vi "SR Scan.vi"() -> ()   [LabVIEW 2014]
uses:
  user.lib/SpectralRadar.llb/LabVIEW Helper.lvlib
  <vilib>/Utility/error.llb/DialogType.ctl
  user.lib/SpectralRadar.llb/OCT Device.lvclass
  user.lib/SpectralRadar.llb/Processing.lvclass
  user.lib/SpectralRadar.llb/Probe.lvclass
  user.lib/SpectralRadar.llb/FullRange.lvclass
  user.lib/SpectralRadar.llb/Settings.lvclass
  user.lib/SpectralRadar.llb/FileSelection.lvlib
  user.lib/SpectralRadar.llb/Scan Pattern.lvclass
  user.lib/SpectralRadar.llb/Raw Data.lvclass
  user.lib/SpectralRadar.llb/Data.lvclass
  user.lib/SpectralRadar.llb/display Data 1D in XY-Graph.vi
  user.lib/SpectralRadar.llb/Normal Direction Selection.ctl
  user.lib/SpectralRadar.llb/Colored Data.lvclass
  user.lib/SpectralRadar.llb/Buffer.lvclass
  user.lib/SpectralRadar.llb/Coloring.lvclass
  user.lib/SpectralRadar.llb/Colored Data Export Format Selection.ctl
  user.lib/SpectralRadar.llb/Probe Parameter Int Selection.ctl
  user.lib/SpectralRadar.llb/Processing Parameter Int Selection.ctl
  user.lib/SpectralRadar.llb/ImageField.lvclass
  user.lib/SpectralRadar.llb/display Data 2D.vi
  user.lib/SpectralRadar.llb/Post Processing.lvlib
  user.lib/SpectralRadar.llb/Raw Data Export Format Selection.ctl
  user.lib/SpectralRadar.llb/Data Analyzation Selection.ctl
  user.lib/SpectralRadar.llb/Coloring Byteorder.ctl
  user.lib/SpectralRadar.llb/set Scan Output.vi
  user.lib/SpectralRadar.llb/Data Export Format Selection.ctl
  user.lib/SpectralRadar.llb/Colorscheme Selection.ctl
panel:
  in  "Average A-scan":bool
  in  "Boolean 2":bool
  in  "Filter Options":bool
  in  "Filter":bool
  in  "B-Scan \nAveraging":i32=1 min=1 max=20 step=1
  in  "BScan angle \n[deg]":dbl(knob) scale=0.0..180.0 scale format="%#.6g"
  in  "BScan\nY offset [mm]":dbl min=-5.0 max=5.0 format="%_4f"
  in  "BScan\nX offset [mm]":dbl min=-5.0 max=5.0 format="%_4f"
  out "ImageField":refnum<class "ImageField.lvclass">
  in  "Auto Range Button":bool
  in  "Image field correction":bool
  out "Save All Progress":i32(slide) min=0 max=35 scale=0.0..11.0
  in  "Palette":T1
  in  "Light":dbl(slide)=51.27999885380268 caption="Sharpness" min=0.0 max=100.0 step=0.009999999776482582 scale=0.0..100.0
  out "Coloring":refnum<class "Coloring.lvclass">
  out "GalvoControl":refnum<class "Probe.lvclass">
  out "Scan Pattern":refnum<class "Scan Pattern.lvclass">
  out "AutoSafe":bool
  in  "Stability":dbl(slide) caption="SNR" min=0.0 max=1.0 step=1.0
  in  "Averaging*Binning":i32(slide)=1 caption="Quality" min=1 max=200 step=1 scale=1.0..200.0
  in  "Options":bool
  in  "Window":T2(ring)
  in  "ShowVideoImage":bool=TRUE caption="Show Video Image"
  out "StreamingPath":path
  in  "Streaming":bool caption="Stream B-Scans"
  out "Image":T3(plugin-control)
  out "Frame Rate":dbl=6.134969234466553 format="%#_3g"
  in  "RunMeasurement":bool
  out "StopIndicator":bool
  in  "Save all":bool
  in  "Brightness":sgl(slide)=0.5272727 caption="Sharpness" min=0 max=1 step=0.01 scale=0.0..1.0
  in  "Contrast":sgl(slide)=0.53333336 caption="Sharpness" min=0 max=1 step=0.01 scale=0.0..1.0
  in  "Saturation":sgl(slide)=0.5212121 caption="Sharpness" min=0 max=1 step=0.01 scale=0.0..1.0
  out "Spacing Z":dbl=2.0 min=1.0 max=500.0 step=1.0 format="%-#2_3f"
  in  "Save":bool
  in  "Description":string
  in  "LowerBScanBorder":dbl=0.972000002861023 min=1.4420210526315789 max=4.806736842105263 step=0.1 format="%.2f"
  in  "UpperBScanBorder":dbl min=0.0 max=0.9613473684210526 step=0.10000000149011612 format="%.2f"
  out "Reference Intensity":sgl(slide) max=140000 scale=0.0..1.0
  out "Next File Name":path=path "D:/OCTData"
  in  "Set Path":bool
  in  "Recallibrate":bool
  in  "Range X [mm]":dbl=2.0 caption="Bereich [mm]" min=0.0 max=10.0 step=0.5 format="%_3f"
  out "Spacing X [µm]":dbl=2.0 min=1.0 max=500.0 step=1.0 format="%#_3g"
  in  "Columns":i32=1000 min=50 max=10240 step=1
  in  "Cursors":bool
  out "Cursor on":bool
  in  "Index of Refraction":dbl=1.0 min=1.0 max=5.0 step=0.10000000149011612 format="%.3f"
  out "Distance Y [mm]":sgl format="%.3f"
  out "Distance X [mm]":sgl format="%.3f"
  out "AScan":cluster{"B-Scan":sgl[], i32[]}(graph)
  in  "Image#":i32=1 caption="of 0" min=1 max=1 step=1
  in  "QuitApp":bool
  in  "Boundries":cluster{sgl, sgl}(slide)={76.65738, 42.00557} scale=15.0..120.0
  out "B-Scan":sgl[][](graph)
  # "Version 5.0"
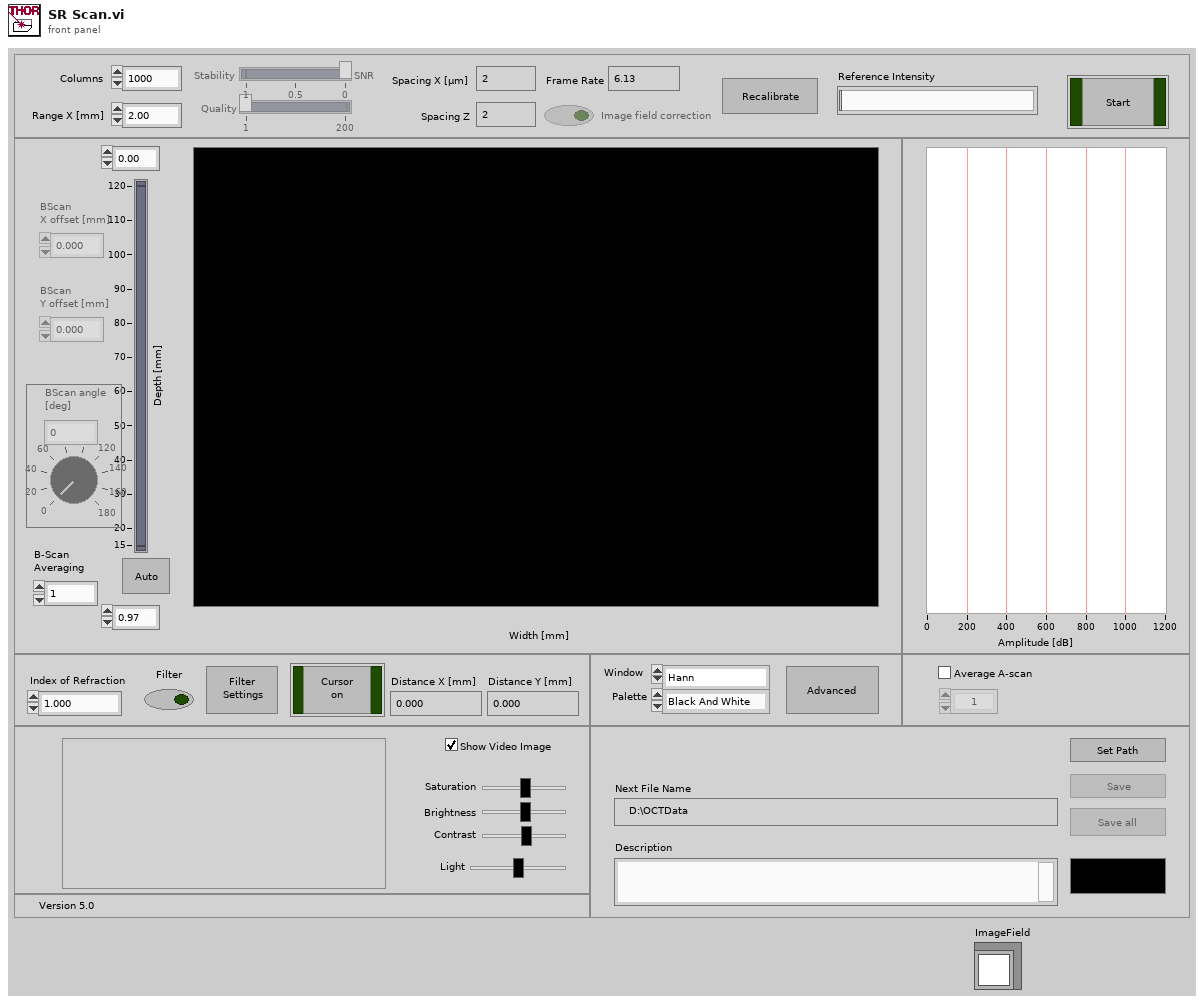
[diagram p1: front panel]
types:
  T1 = typedef "Coloring.lvclass/Colorscheme Selection.ctl" = enum16{"Black And White", "Inverted Black And White", "Color", "Black and Orange", "Black and Red", "Doppler Phase Coloring"}
  T2 = enum16{"Hann", "Hamming", "Gauss", "Tapered Cosine", "Blackman", "4 Term B-Harris"}
  T3 = typedef "IMAQ Image.ctl" = refnum<image>
  T4 = typedef "Coloring.lvclass/Coloring Byteorder.ctl" = enum16{"RGBA32", "BGRA32", "ARGB32", ""}
  T5 = enum16{"Full Well Capacity", "z Spacing", "z Range", "Dynamc Range Min [dB]", "Dynamic Range Low [dB]", "Dynamic Range High [dB]", "Dynamic Range Max [dB]"}
  T6 = typedef "Probe.lvclass/Probe Parameter Int Selection.ctl" = enum16{"Apodization Cycles", "Oversampling", "Oversampling Slow Axis", "Speckle Reduction"}
  T7 = typedef "Processing.lvclass/Processing Parameter Int Selection.ctl" = enum32{"Spectrum Averaging", "A-Scan Averaging", "B-Scan Averaging", "Zero Padding", "Number of Threads", "Fourier Averaging"}
  T8 = typedef "Data.lvclass/Normal Direction Selection.ctl" = enum16{"Direction 1", "Direction 2", "Direction 3"}
  T9 = typedef "Data.lvclass/Data Export Format Selection.ctl" = enum16{"SRM (Spectral Radar Metafile)", "RAW", "CSV", "TXT", "Table TXT", "Fits", "VFF", "VTK", "TIFF"}
  T10 = typedef "Colored Data.lvclass/Colored Data Export Format Selection.ctl" = enum16{"SRM (Spectral Radar Metafile)", "RAW", "BMP", "PNG", "JPG", "PDF", "TIFF"}
  T11 = enum16{"Asynchronous Continuous", "Asynchronous Finite", "Synchronous"}
  T12 = typedef "Data.lvclass/Data Analyzation Selection.ctl" = enum16{"Min", "Mean", "Max"}
  T13 = typedef "Raw Data.lvclass/Raw Data Export Format Selection.ctl" = enum16{"RAW", "SRR (Spectral Radar Raw)"}
  T14 = typedef "DialogType.ctl" = u16
  T15 = typedef "Image Type" = u32
  T16 = enum8{"Enabled", "Disabled", "Disabled and Grayed Out"}
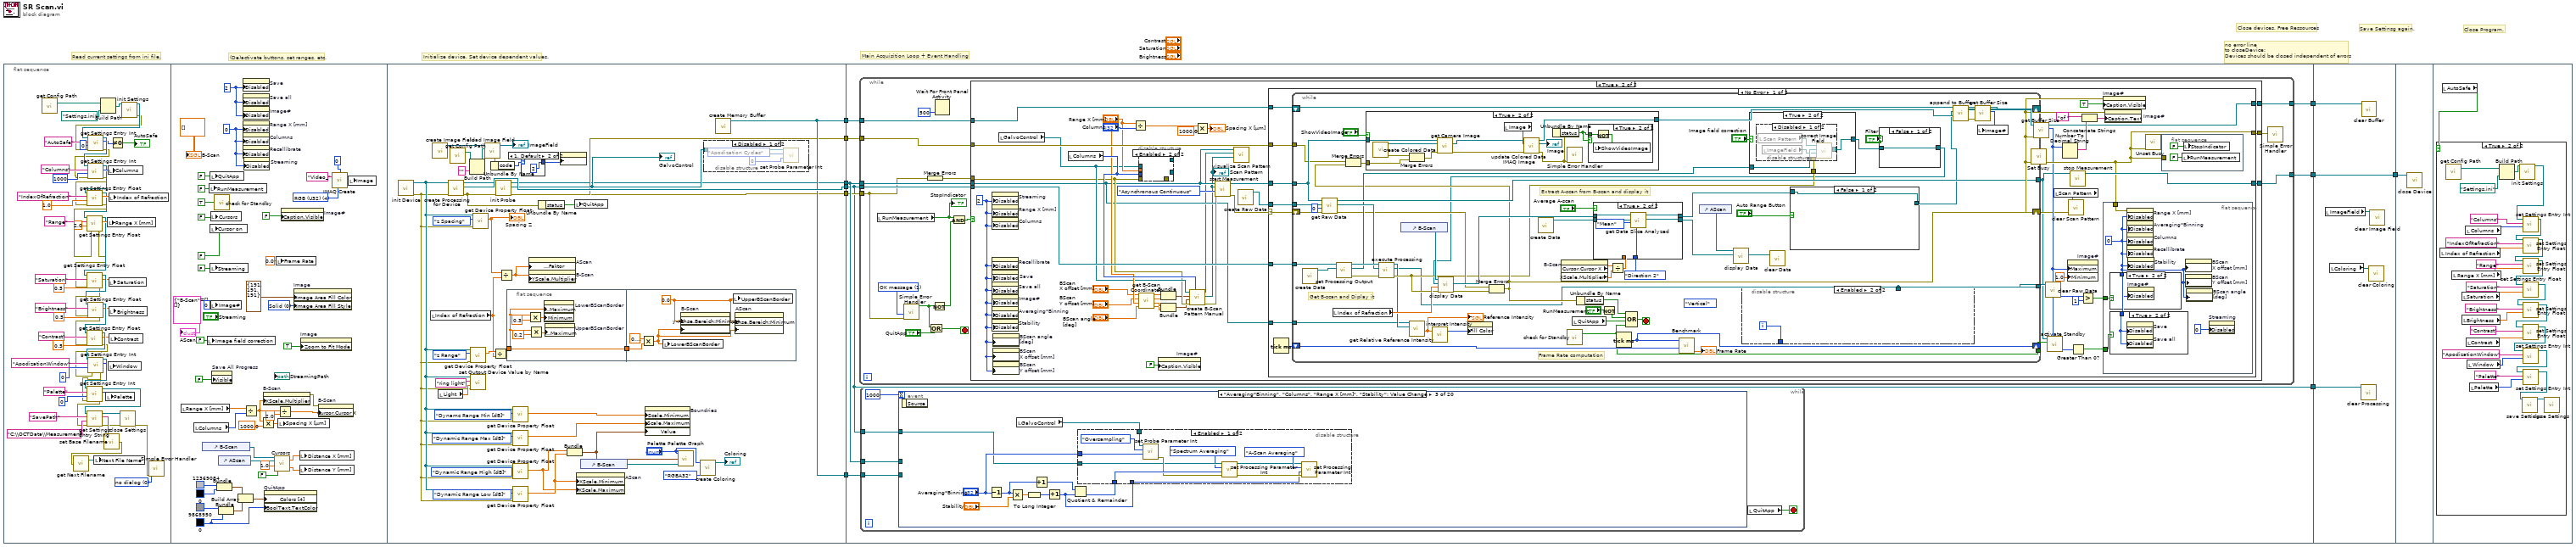
[diagram p0: block diagram]
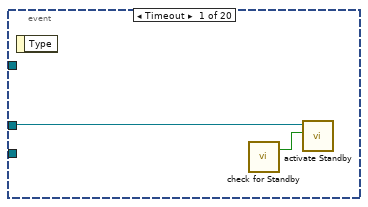
[diagram p4: hidden frame]
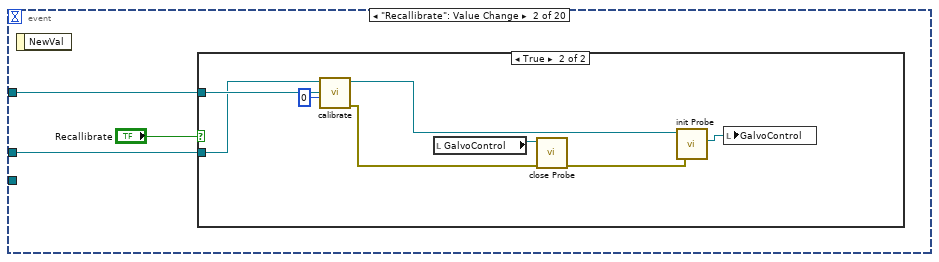
[diagram p5: hidden frame]
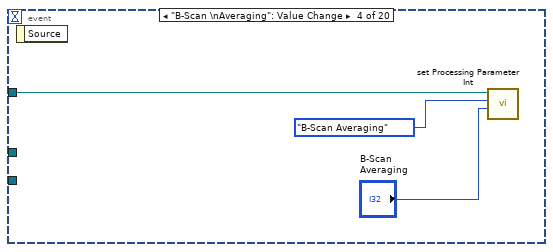
[diagram p8: hidden frame]
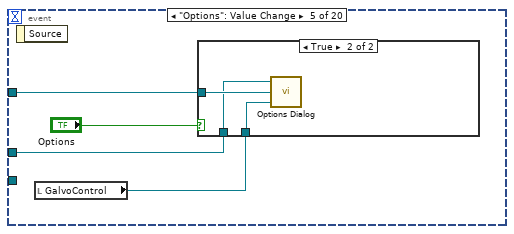
[diagram p9: hidden frame]
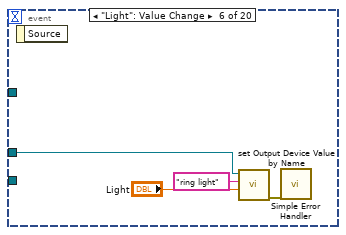
[diagram p11: hidden frame]
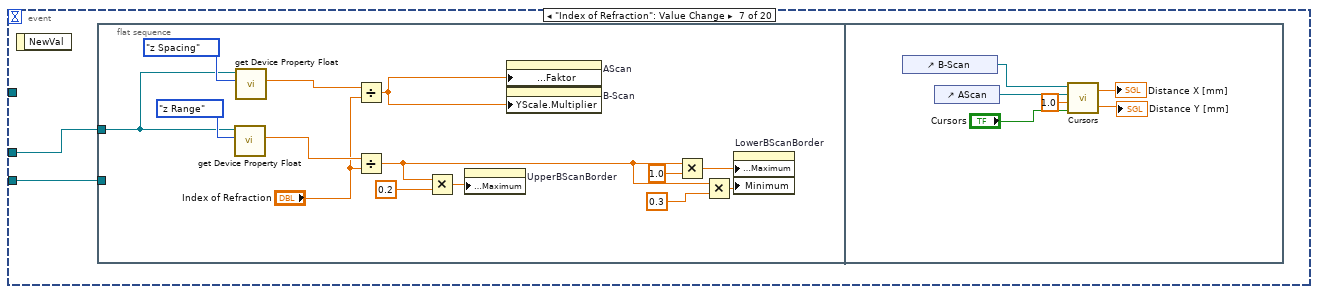
[diagram p12: hidden frame]
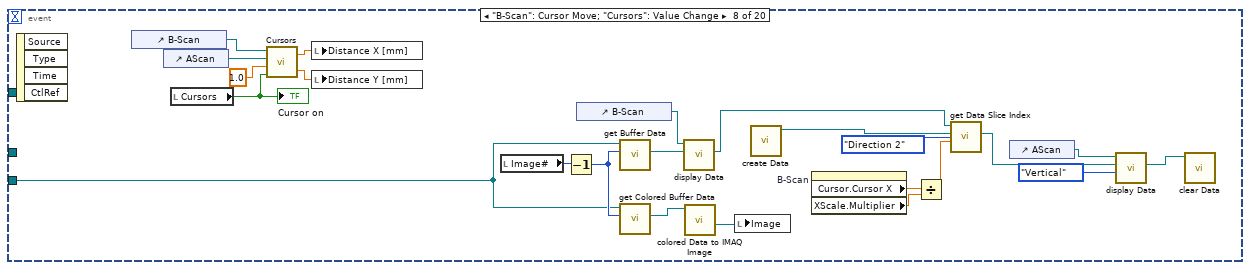
[diagram p13: hidden frame]
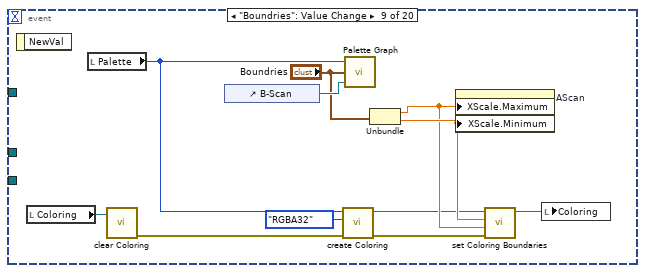
[diagram p14: hidden frame]
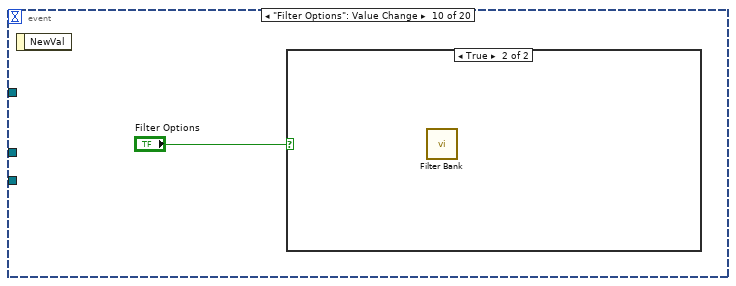
[diagram p15: hidden frame]
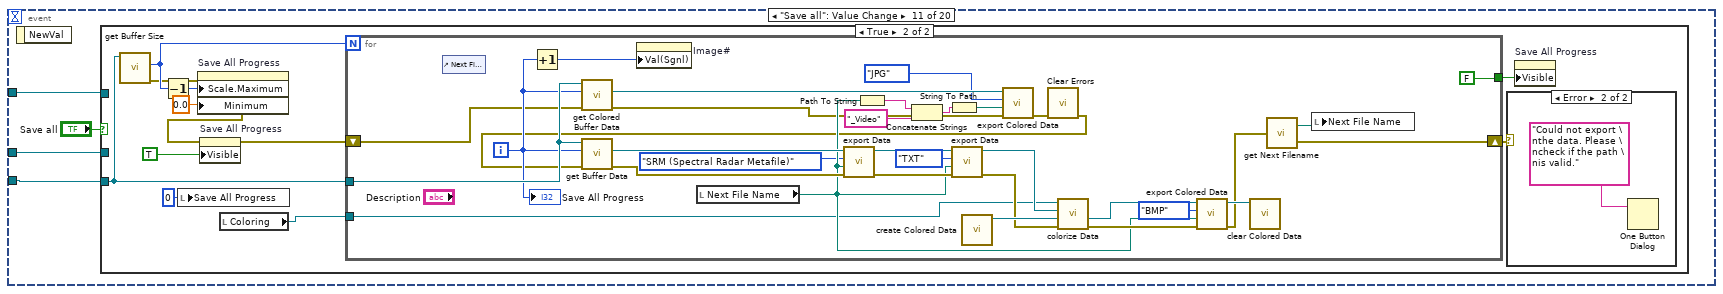
[diagram p17: hidden frame]
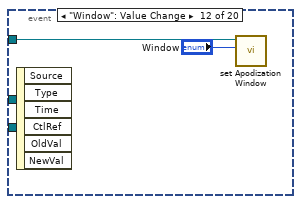
[diagram p20: hidden frame]
diagram:
  # "Close Program."
  # "Save Settinsg again."
  # "Close devices, Free Ressources"
  # "Main Acquisition Loop + Event Handling"
  # "Initialize device. Set device dependent values."
  # "(De)activate buttons, set ranges, etc."
  # "Read current settings from ini file."
  # "no error line\nto closeDevice:\nDevices should be closed independent of errors"
  n1 = flat-sequence {
    tunnel: [w114] -> w10
    tunnel: [w116] -> w7
    tunnel: [w151] -> w6
    tunnel: [w115] -> w4
    tunnel: [w140] -> w3
    tunnel: [w140] -> w1
    tunnel: w10 -> [w175]
    tunnel: [w176] -> w8
    tunnel: w7 -> [w174]
    tunnel: w6 -> [w172]
    tunnel: [w172] -> w5
    tunnel: w4 -> [w173]
    tunnel: w3 -> [w171]
    tunnel: [w170] -> w2
    tunnel: w1 -> [w169]
    tunnel: [w668] -> w9
    tunnel: w8 -> [w668]
    tunnel: w5 -> [w667]
    tunnel: w2 -> [w666]
    tunnel: w9 -> [w669]
    frame #0 {
      w22 = T14 0 items=["no dialog", "OK message", "continue or stop message", "OK message + warnings", "continue/stop + warnings"] ("type of dialog (OK msg:1)")
      n2 = call "get Config Path.vi"() -> ("Path"=w25:path)  [unwired: 1 in, 1 out]
      n3 = Build Path(base path=w25, name or relative path=path "Settings.ini" ("Relative \"SpectralRadar.ini\" Path")) -> (appended path=w69:path)
      n4 = call "init Settings.vi"("Path to settings file"=w69) -> ("error out"=w24:errorcluster, "Settings"=w56:refnum<class "Settings.lvclass">)  [unwired: 5 in]
      n5 = call "get Settings Entry Int.vi"("error in (no error)"=w24, "Default Value"=0, "Node Name"="AutoSafe", "Settings"=w56) -> ("error out"=w19:errorcluster, "Value"=w53:i32, "Settings"=w57:refnum<class "Settings.lvclass">)  [unwired: 1 in]
      n6 = call "get Settings Entry Int.vi"("error in (no error)"=w19, "Default Value"=1000, "Node Name"="Columns", "Settings"=w57) -> ("error out"=w18:errorcluster, "Value"=w67:i32, "Settings"=w59:refnum<class "Settings.lvclass">)  [unwired: 1 in]
      n7 = call "get Settings Entry Float.vi"("error in (no error)"=w18, "Default Value"=1.0, "Node Name"="IndexOfRefraction", "Settings"=w59) -> ("error out"=w17:errorcluster, "Value"=w63:dbl, "Settings"=w58:refnum<class "Settings.lvclass">)  [unwired: 1 in]
      n8 = call "get Settings Entry Float.vi"("error in (no error)"=w17, "Default Value"=2.0, "Node Name"="Range", "Settings"=w58) -> ("error out"=w16:errorcluster, "Value"=w60:dbl, "Settings"=w49:refnum<class "Settings.lvclass">)  [unwired: 1 in]
      n9 = call "get Settings Entry Float.vi"("error in (no error)"=w16, "Default Value"=0.5, "Node Name"="Saturation", "Settings"=w49) -> ("error out"=w15:errorcluster, "Value"=w35:dbl, "Settings"=w46:refnum<class "Settings.lvclass">)  [unwired: 1 in]
      n10 = call "get Settings Entry Float.vi"("error in (no error)"=w15, "Default Value"=0.5, "Node Name"="Brightness", "Settings"=w46) -> ("error out"=w14:errorcluster, "Value"=w34:dbl, "Settings"=w39:refnum<class "Settings.lvclass">)  [unwired: 1 in]
      n11 = call "get Settings Entry Float.vi"("error in (no error)"=w14, "Default Value"=0.5, "Node Name"="Contrast", "Settings"=w39) -> ("error out"=w13:errorcluster, "Value"=w33:dbl, "Settings"=w38:refnum<class "Settings.lvclass">)  [unwired: 1 in]
      n12 = call "get Settings Entry Int.vi"("error in (no error)"=w13, "Default Value"=0, "Node Name"="ApodizationWindow", "Settings"=w38) -> ("error out"=w12:errorcluster, "Value"=w36:i32, "Settings"=w37:refnum<class "Settings.lvclass">)  [unwired: 1 in]
      n13 = call "get Settings Entry Int.vi"("error in (no error)"=w12, "Default Value"=0, "Node Name"="Palette", "Settings"=w37) -> ("error out"=w11:errorcluster, "Value"=w20:i32, "Settings"=w31:refnum<class "Settings.lvclass">)  [unwired: 1 in]
      n14 = call "get Settings Entry String.vi"("error in (no error)"=w11, "Default Value"="C:\\OCTData\\Measurement", "Node Name"="SavePath", "Settings"=w31) -> ("error out"=w23:errorcluster, "Value"=w28:string, "Settings"=w30:refnum<class "Settings.lvclass">)  [unwired: 1 in]
      n15 = call "set Base Filename.vi"("Base"=w28) -> ("error out"=w27:errorcluster)  [unwired: 1 in]
      n16 = call "get Next Filename.vi"("error in (no error)"=w27) -> ("Next File Name"=w26:path)  [unwired: 1 out]
      n17 = local write "Next File Name"(w26) -> ()
      n18 = local write "Palette"(w20) -> ()
      n19 = local write "Range X [mm]"(w60) -> ()
      n20 = local write "Columns"(w67) -> ()
      n21 = local write "Window"(w36) -> ()
      n22 = local write "Index of Refraction"(w63) -> ()
      n23 = local write "Saturation"(w35) -> ()
      n24 = local write "Brightness"(w34) -> ()
      n25 = local write "Contrast"(w33) -> ()
      n26 = Not Equal To 0?(x=w53) -> (x != 0?=→"AutoSafe":bool)
      n27 = call "close Settings.vi"("error in (no error)"=w23, "Settings"=w30) -> ("error out"=w21:errorcluster)  [unwired: 5 in]
      n28 = call <vilib>:"Simple Error Handler.vi"("type of dialog (OK msg:1)"=w22, "error in (no error)"=w21) -> ()  [unwired: 3 in, 5 out]
    }
    frame #1 {
      w77 = T15 4 items=["Grayscale (U8)", "Grayscale (I16)", "Grayscale (SGL)", "Complex (CSG)", "RGB (U32)", "HSL (U32)", "RGB (U64)", "Grayscale (U16)"] ("Image Type")
      w83 = u32 0 items=["Default"=3, "Solid"=0, "Hatch"=2] ("Image Area:Background:Fill Style")
      w104 = u32 0
      w112 = u8 0 ("Deaktiviert")
      w113 = u8 2 ("Deaktiviert")
      n29 = local read "Range X [mm]"() -> (w90:dbl)
      n30 = local read "Columns"() -> (w85:i32)
      n31 = control-ref of="B-Scan"() -> (w93:refnum<vi>)
      n32 = local write "Image field correction"(FALSE ("Confocal correction")) -> ()
      n33 = local write "RunMeasurement"(FALSE ("s/t")) -> ()
      n34 = local write "QuitApp"(FALSE ("QuitApp")) -> ()
      n35 = local write "Cursor on"(FALSE ("Cursor on")) -> ()
      n36 = local write "Streaming"(FALSE ("Streaming")) -> ()
      n37 = local write "Cursors"(FALSE ("Cursors")) -> ()
      n38 = local write "Image#"(0 ("Image#")) -> ()
      n39 = property on="Save All Progress" class="Slide (strict)"("Visible"=FALSE) -> ()  [unwired: 2 in, 2 out]
      n40 = call "check for Standby.vi"("ResetTimer"=TRUE) -> ()  [unwired: 2 out]
      n41 = Bundle(u32 12369084, u32 0) -> (w101:cluster{u32, u32})  [unwired: 1 in]
      n42 = control-ref of="AScan"() -> (w94:refnum<vi>)
      n43 = Bundle(u32 9868950, w104) -> (w102:cluster{u32, u32})  [unwired: 1 in]
      n44 = Build Array(w101, w102) -> (w103:cluster{u32, u32}[])
      n45 = property on="Save" class="Bool"("Disabled"=w113) -> ()  [unwired: 2 in, 2 out]
      n46 = property on="Save all" class="Bool (strict)"("Disabled"=w113) -> ()  [unwired: 2 in, 2 out]
      n47 = property on="Image#" class="DigNum (strict)"("Disabled"=w113) -> ()  [unwired: 2 in, 2 out]
      n48 = property on="Range X [mm]" class="DigNum (strict)"("Disabled"=w112) -> ()  [unwired: 2 in, 2 out]
      n49 = property on="Columns" class="DigNum (strict)"("Disabled"=w112) -> ()  [unwired: 2 in, 2 out]
      n50 = property on="Recallibrate" class="Bool"("Disabled"=w112) -> ()  [unwired: 2 in, 2 out]
      n51 = property on="Streaming" class="Bool (strict)"("Disabled"=w112) -> ()  [unwired: 2 in, 2 out]
      n52 = Divide(x=w90, y=w85) -> (x/y=w88:dbl)
      n53 = Multiply(x=w88, y=1000.0) -> (x*y=w86:dbl)
      n54 = property on="B-Scan" class="IntGraph (strict)"("XScale.Multiplier"=w88) -> (error out=w91:errorcluster)  [unwired: 2 in, 1 out]
      n55 = property on="QuitApp" class="Bool (strict)"("Colors [4]"=w103, "BoolText.TextColor"=w104) -> ()  [unwired: 2 in, 2 out]
      n56 = call "Cursors.vi"("Cursors"=FALSE, "IndexOfRefraction"=sgl 1.0, "ReferenceAScan"=w94, "ReferenceBScan"=w93) -> ("DistanceZ"=w97:sgl, "DistanceX"=w96:sgl)
      n57 = local write "Frame Rate"(0.0 ("Frame Rate")) -> ()
      n58 = Divide(x=w88, y=2.0) -> (x/y=w87:dbl)
      n59 = local write "Spacing X [µm]"(w86) -> ()
      n60 = property on="Image#" class="DigNum (strict)"("Caption.Visible"=FALSE ("Untertitel.Sichtbar")) -> ()  [unwired: 2 in, 2 out]
      n61 = property on="Image" class="ImageControl"("Image Area Fill Color"=cluster{"Red":u8, "Green":u8, "Blue":u8} {"Red"=191, "Green"=191, "Blue"=191} ("Image Area:Background:Fill Color"), "Image Area Fill Style"=w83) -> ()  [unwired: 2 in, 2 out]
      n62 = local write "Distance X [mm]"(w96) -> ()
      n63 = local write "Distance Y [mm]"(w97) -> ()
      n64 = property on="Image" class="ImageControl"("Zoom to Fit Mode"=TRUE) -> ()  [unwired: 2 in, 2 out]
      n65 = property on="B-Scan" class="IntGraph (strict)"(error in=w91, "Cursor.Cursor X"=w87) -> ()  [unwired: 1 in, 2 out]
      n66 = call "IMAQ Create"("Border Size"=0, "Image Name"="Video_", "Image Type"=w77) -> ("New Image"=w79:T3)  [unwired: 2 in, 1 out]
      n67 = local write "Image"(w79) -> ()
      "B-Scan" <- sgl[][] [] ("B-Scan")
      "AScan" <- cluster{"B-Scan":sgl[], i32[]} {"B-Scan"=[], []} ("AScan")
    }
    frame #2 {
      n68 = call "init Device.vi"() -> ("error out"=w118:errorcluster, "OCTDevice"=w124:refnum<class "OCT Device.lvclass">)  [unwired: 6 in]
      n69 = local read "Index of Refraction"() -> (w133:dbl)
      n70 = call "create Image Field.vi"() -> ("ImageField out"=w129:refnum<class "ImageField.lvclass">)  [unwired: 6 in, 1 out]
      n71 = local read "Light"() -> (w130:dbl)
      n72 = call "create Processing for Device.vi"("error in (no error)"=w118, "OCTDevice"=w124) -> ("error out"=w116:errorcluster, "Processing"=w151:refnum<class "Processing.lvclass">, "OCTDevice"=w138:refnum<class "OCT Device.lvclass">)  [unwired: 3 in]
      n73 = call "get Config Path.vi"() -> ("Path"=w128:path)  [unwired: 1 in, 1 out]
      n74 = Build Path(base path=w128, name or relative path="") -> (appended path=w126:path)
      n75 = call "get Device Property Float.vi"("error in (no error)"=w118, "Device Property Float Selection"=T5."z Range", "OCTDevice"=w124) -> ("Value"=w136:dbl)  [unwired: 2 in, 2 out]
      n76 = call "set Output Device Value by Name.vi"("error in (no error)"=w118, "Value"=w130, "Identifier"="ring light", "OCTDevice"=w124) -> ()  [unwired: 2 in, 2 out]
      n77 = call "get Device Property Float.vi"("error in (no error)"=w118, "Device Property Float Selection"=T5."z Spacing", "OCTDevice"=w124) -> ("Value"=w134:dbl)  [unwired: 2 in, 2 out]
      "Spacing Z" <- w134
      n78 = call "load Image Field.vi"("Path"=w126, "ImageField in"=w129) -> ("error out"=w123:errorcluster, "ImageField out"=→"ImageField":refnum<class "ImageField.lvclass">)  [unwired: 4 in]
      n79 = Unbundle By Name(w123) -> ("code"=w122:i32)
      n80 = Divide(x=w136, y=w133) -> (x/y=w132:dbl)
      n81 = call "init Probe.vi"("error in (no error)"=w116, "OCT Device [In]"=w138) -> ("error out"=w115:errorcluster, "GalvoControl"=w117:refnum<class "Probe.lvclass">, "OCT Device [Out]"=w114:refnum<class "OCT Device.lvclass">)  [unwired: 3 in]
      "GalvoControl" <- w117
      n82 = Divide(x=w134, y=w133) -> (x/y=w135:dbl)
      n83 = flat-sequence {
        tunnel: w132 -> [w158]
        tunnel: [w158] -> w120
        tunnel: w120 -> [w163]
        frame #0 {
          n84 = Multiply(x=w158, y=0.3) -> (x*y=w162:dbl)
          n85 = Multiply(x=w158, y=0.2) -> (x*y=w160:dbl)
          n86 = property on="LowerBScanBorder" class="DigNum (strict)"("Wertebereich:Maximum"=w158, "Minimum"=w162) -> ()  [unwired: 2 in, 2 out]
          n87 = property on="UpperBScanBorder" class="DigNum (strict)"("Wertebereich:Maximum"=w160) -> ()  [unwired: 2 in, 2 out]
        }
        frame #1 {
          w165 = 0.0 ("y")
          n88 = Multiply(x=0.800000011920929, y=w163) -> (x*y=w166:dbl)
          n89 = local write "LowerBScanBorder"(w166) -> ()
          n90 = property on="B-Scan" class="IntGraph (strict)"("y-Achse.Bereich:Minimum"=w165, "y-Achse.Bereich:Maximum"=w166) -> ()  [unwired: 2 in, 2 out]
          n91 = local write "UpperBScanBorder"(w165) -> ()
          n92 = property on="AScan" class="XYGraph (strict)"("y-Achse.Bereich:Minimum"=w165, "y-Achse.Bereich:Maximum"=w166) -> ()  [unwired: 2 in, 2 out]
        }
      }
      n93 = call "get Device Property Float.vi"("error in (no error)"=w118, "Device Property Float Selection"=T5."Dynamc Range Min [dB]", "OCTDevice"=w124) -> ("Value"=w150:dbl)  [unwired: 2 in, 2 out]
      n94 = call "get Device Property Float.vi"("error in (no error)"=w118, "Device Property Float Selection"=T5."Dynamic Range Max [dB]", "OCTDevice"=w124) -> ("Value"=w149:dbl)  [unwired: 2 in, 2 out]
      n95 = call "get Device Property Float.vi"("error in (no error)"=w118, "Device Property Float Selection"=T5."Dynamic Range High [dB]", "OCTDevice"=w124) -> ("Value"=w141:dbl)  [unwired: 2 in, 2 out]
      n96 = call "get Device Property Float.vi"("error in (no error)"=w118, "Device Property Float Selection"=T5."Dynamic Range Low [dB]", "OCTDevice"=w124) -> ("Value"=w142:dbl)  [unwired: 2 in, 2 out]
      n97 = case shown="1, Default" w122 {
        selector: w122 -> [w167 _]
        tunnel: [w167 2 ("code")] -> w121
        frame 0 {
        }
        frame 1, Default {
        }
      }
      n98 = property on="AScan" class="XYGraph (strict)"("y-Achse.Offset und Faktor:Faktor"=w135) -> ()  [unwired: 2 in, 2 out]
      n99 = property on="B-Scan" class="IntGraph (strict)"("YScale.Multiplier"=w135) -> ()  [unwired: 2 in, 2 out]
      n100 = Unbundle By Name(w116) -> ("status"=w152:bool)
      n101 = property on="Image field correction" class="Bool (strict)"("DisabledEnum"=w121) -> ()  [unwired: 2 in, 2 out]
      n102 = Bundle("Value"=w141, "Value"=w142) -> (w154:cluster{"Value":dbl, "Value":dbl})  [unwired: 1 in]
      n103 = local write "QuitApp"(w152) -> ()
      n104 = property on="AScan" class="XYGraph (strict)"("XScale.Minimum"=w142, "XScale.Maximum"=w141) -> ()  [unwired: 2 in, 2 out]
      n105 = control-ref of="B-Scan"() -> (w153:refnum<vi>)
      n106 = property on="Boundries" class="Slide (strict)"("Scale.Minimum"=w150, "Scale.Maximum"=w149, "Value"=w154) -> ()  [unwired: 2 in, 2 out]
      n107 = call "Palette Graph.vi"("Reference to the B-scan Graph"=w153, "Boundaries"=w154, "Color Scheme"="Palette") -> ()
      n108 = call "create Coloring.vi"("Color Byte Order"=Coloring_Byteorder."RGBA32", "Color Table Selection"="Palette") -> ("Coloring"=→"Coloring":refnum<class "Coloring.lvclass">)  [unwired: 4 in, 1 out]
      n109 = disable-structure shown="Disabled" {
        disable-tunnel: w117 -> [w157 _]
        frame Disabled {
          n110 = call "set Probe Parameter Int.vi"("Value"=0, "Probe Parameter Int"=Probe_Parameter_Int_Selection."Apodization Cycles", "GalvoControl"=w157) -> ()  [unwired: 3 in, 2 out]
        }
        frame Enabled {
        }
      }
      n111 = call "create Memory Buffer.vi"() -> ("Buffer"=w140:refnum<class "Buffer.lvclass">)  [unwired: 6 in, 1 out]
    }
    frame #3 {
      n112 = while {
        tunnel: w175 -> [w457]
        tunnel: [w456] -> w176
        tunnel: w174 -> [w455]
        tunnel: w172 -> [w454]
        tunnel: w173 -> [w445]
        tunnel: w171 -> [w449]
        tunnel: [w448] -> w170
        stop <- w459 stop-if-true
        w447 = T14 1 items=["no dialog", "OK message", "continue or stop message", "OK message + warnings", "continue/stop + warnings"] ("type of dialog (OK msg:1)")
        n113 = local read "RunMeasurement"() -> (w452:bool)
        "StopIndicator" <- w452
        n114 = call <vilib>:"Simple Error Handler.vi"("type of dialog (OK msg:1)"=w447, "error in (no error)"=w445) -> ("error?"=w451:bool)  [unwired: 3 in, 4 out]
        n115 = Merge Errors(w445) -> (w446:errorcluster)
        n116 = Or(x=w451, y="QuitApp") -> (x .or. y?=w459:bool)
        n117 = Not(x=w451) -> (.not. x?=w450:bool)
        n118 = Wait For Front Panel Activity(1:500 ("Timeout in ms (-1 kein Timeout)")) -> ()  [unwired: 2 in, 1 out]
        n119 = And(x=w452, y=w450) -> (x .and. y?=w453:bool)
        n120 = case shown="True" w453 {
          tunnel: [w462 w497] -> w461
          tunnel: w457 -> [w464 w468]
          tunnel: [w464 w490] -> w456
          tunnel: w455 -> [_ w489]
          tunnel: w454 -> [_ w488]
          tunnel: w449 -> [w463 w484]
          tunnel: [w463 w483] -> w448
          tunnel: w446 -> [w462 w477]
          frame False {
          }
          frame True {
            w479 = u8 2 ("Deaktiviert")
            n121 = property on="Streaming" class="Bool (strict)"("Disabled"=w479) -> ()  [unwired: 2 in, 2 out]
            n122 = property on="Range X [mm]" class="DigNum (strict)"("Disabled"=w479) -> ()  [unwired: 2 in, 2 out]
            n123 = property on="Columns" class="DigNum (strict)"("Disabled"=w479) -> ()  [unwired: 2 in, 2 out]
            n124 = property on="Recallibrate" class="Bool"("Disabled"=w479) -> ()  [unwired: 2 in, 2 out]
            n125 = property on="Save" class="Bool"("Disabled"=w479) -> ()  [unwired: 2 in, 2 out]
            n126 = property on="Save all" class="Bool (strict)"("Disabled"=w479) -> ()  [unwired: 2 in, 2 out]
            n127 = property on="Image#" class="DigNum (strict)"("Disabled"=w479) -> ()  [unwired: 2 in, 2 out]
            n128 = property on="Averaging*Binning" class="Slide (strict)"("Disabled"=w479) -> ()  [unwired: 2 in, 2 out]
            n129 = property on="Stability" class="Slide (strict)"("Disabled"=w479) -> ()  [unwired: 2 in, 2 out]
            n130 = property on="BScan angle \n[deg]" class="Knob (strict)"("DisabledEnum"=w479) -> ()  [unwired: 2 in, 2 out]
            n131 = property on="BScan\nX offset [mm]" class="DigNum (strict)"("DisabledEnum"=w479) -> ()  [unwired: 2 in, 2 out]
            n132 = property on="BScan\nY offset [mm]" class="DigNum (strict)"("DisabledEnum"=w479) -> ()  [unwired: 2 in, 2 out]
            n133 = local read "GalvoControl"() -> (w478:refnum<class "Probe.lvclass">)
            n134 = local read "Columns"() -> (w482:i32)
            n135 = Divide(x="Range X [mm]", y="Columns") -> (x/y=w494:dbl)
            n136 = disable-structure shown="Enabled" {
              disable-tunnel: "Range X [mm]" -> [w504 _]
              disable-tunnel: [w503 _] -> _
              disable-tunnel: w478 -> [w502 _]
              disable-tunnel: [w501 _] -> _
              disable-tunnel: [w500 _] -> _
              disable-tunnel: w477 -> [w499 _]
              disable-tunnel: w482 -> [w498 _]
              frame Disabled {
                n137 = call "create B-Scan Pattern.vi"("Probe"=w502, "Range"=w504, "AScans"=w498, "error in (no error)"=w499) -> ("Probe"=w500:refnum<class "Probe.lvclass">, "Scan Pattern"=w501:refnum<class "Scan Pattern.lvclass">, "error out"=w503:errorcluster)  [unwired: 1 in]
              }
              frame Enabled {
              }
            }
            n138 = call "get B-Scan Coordinates.vi"("BScan Angle [deg]"="BScan angle \n[deg]", "BScan Range"="Range X [mm]", "Offset Y"="BScan\nY offset [mm]", "Offset X"="BScan\nX offset [mm]") -> ("End Y"=w473:dbl, "End X"=w474:dbl, "Start Y"=w475:dbl, "Start X"=w476:dbl)
            n139 = property on="Image#" class="DigNum (strict)"("Caption.Visible"=FALSE ("Untertitel.Sichtbar")) -> ()  [unwired: 2 in, 2 out]
            n140 = Bundle("Start X"=w476, "Start Y"=w475) -> (w472:cluster{"Start X":dbl, "Start Y":dbl})  [unwired: 1 in]
            n141 = Bundle("End X"=w474, "End Y"=w473) -> (w471:cluster{"End X":dbl, "End Y":dbl})  [unwired: 1 in]
            n142 = call "create B-Scan Pattern Manual.vi"("AScans"=w482, "error in (no error)"=w477, "Stop"=w471, "Start"=w472, "Probe in"=w478) -> ("error out"=w480:errorcluster, "Scan Pattern"=w466:refnum<class "Scan Pattern.lvclass">, "Probe out"=w467:refnum<class "Probe.lvclass">)  [unwired: 2 in]
            "Scan Pattern" <- w466
            n143 = Multiply(x=w494, y=1000.0) -> (x*y=→"Spacing X [µm]":dbl)
            n144 = call "start Measurement.vi"("error in (no error)"=w480, "Acquisition Type"=T11."Asynchronous Continuous", "Scan Pattern"=w466, "OCTDevice"=w468) -> ("error out"=w486:errorcluster, "OCTDevice"=w496:refnum<class "OCT Device.lvclass">)  [unwired: 1 in, 1 out]
            n145 = call "visualize Scan Pattern.vi"("Scan Pattern in"=w466, "Probe"=w467, "OCT Device"=w468) -> ()  [unwired: 2 in, 4 out]
            n146 = call "create Raw Data.vi"() -> ("Raw Data"=w487:refnum<class "Raw Data.lvclass">)  [unwired: 6 in, 1 out]
            n147 = case shown="No Error" w486 {
              selector: w486 -> [w516 w658]
              tunnel: [w517 w658] -> w497
              tunnel: w489 -> [w530 _]
              tunnel: w496 -> [w529 w662]
              tunnel: [w521 w661] -> w490
              tunnel: w488 -> [w518 _]
              tunnel: w487 -> [w515 _]
              tunnel: w468 -> [w514 _]
              tunnel: w484 -> [w513 w660]
              tunnel: [w511 w660] -> w483
              frame No Error {
                n148 = Tick Count (ms)() -> (millisecond timer value=w520:u32)
                n149 = while {
                  shift-right: [w596] -> _
                  shift-left: w520 -> [w594]
                  tunnel: w529 -> [w588]
                  tunnel: [w586] -> w519
                  tunnel: [w577] -> w505
                  tunnel: w518 -> [w584]
                  shift-right: [w564] -> w506
                  shift-left: w516 -> [w590]
                  tunnel: w515 -> [w587]
                  tunnel: w514 -> [w550]
                  shift-right: [w574] -> w512
                  shift-left: w513 -> [w576]
                  tunnel: [w544] -> w509
                  tunnel: w530 -> [w565]
                  i -> [w543]
                  stop <- w592 stop-if-true
                  (unwired) enum16{"Horiztonal", "Vertical"}."Vertical" ("Orientation")
                  # "Extract A-scan from B-scan and display it"
                  # "Frame Rate computation"
                  # "Get B-scan and Diplay it"
                  n150 = call "create Data.vi"() -> ("Data"=w583:refnum<class "Data.lvclass">)  [unwired: 6 in, 1 out]
                  n151 = call "get Raw Data.vi"("error in (no error)"=w590, "Camera Index"=0, "RawData in"=w587, "OCTDevice in"=w588) -> ("error out"=w567:errorcluster, "RawData out"=w581:refnum<class "Raw Data.lvclass">, "OCTDevice out"=w577:refnum<class "OCT Device.lvclass">)  [unwired: 1 in]
                  n152 = local read "Index of Refraction"() -> (w570:dbl)
                  n153 = call-poly "set Processing Output.vi"("Data"=w583, "Processing"=w584) -> ("error out"=w579:errorcluster, "Data"=w568:refnum<class "Data.lvclass">, "Processing"=w582:refnum<class "Processing.lvclass">)  [unwired: 3 in]
                  n154 = call "execute Processing.vi"("error in (no error)"=w579, "Raw Data"=w581, "Processing"=w582) -> ("error out"=w552:errorcluster, "Raw Data"=w544:refnum<class "Raw Data.lvclass">, "Processing"=w551:refnum<class "Processing.lvclass">)  [unwired: 2 in]
                  n155 = control-ref of="B-Scan"() -> (w580:refnum<vi>)
                  n156 = call "get Relative Reference Intensity.vi"("Processing"=w551, "OCTDevice"=w550) -> ("Relative Reference Intensity"=w549:dbl)  [unwired: 2 in, 3 out]
                  "Reference Intensity" <- w549
                  n157 = call "interpret Intensity.vi"("Intensity"=w549) -> ("Color"=w548:u32)  [unwired: 1 in, 1 out]
                  n158 = property on="Reference Intensity" class="Slide (strict)"("Fill Color"=w548) -> ()  [unwired: 2 in, 2 out]
                  n159 = call "create Data.vi"() -> ("Data"=w563:refnum<class "Data.lvclass">)  [unwired: 6 in, 1 out]
                  n160 = property on="B-Scan" class="IntGraph (strict)"() -> ("Cursor.Cursor X"=w559:dbl, "XScale.Multiplier"=w558:dbl)  [unwired: 2 in, 2 out]
                  n161 = call "check for Standby.vi"() -> ("TimeOut"=w586:bool)  [unwired: 1 in, 1 out]
                  n162 = local read "QuitApp"() -> (w585:bool)
                  n163 = Not(x="RunMeasurement") -> (.not. x?=w593:bool)
                  n164 = Divide(x=w559, y=w558) -> (x/y=w560:dbl)
                  n165 = Tick Count (ms)() -> (millisecond timer value=w596:u32)
                  n166 = call "Benchmark.vi"("TimeStart"=w594, "TimeFinish"=w596) -> ("AverageFrameRate"=→"Frame Rate":sgl)  [unwired: 2 in, 2 out]
                  n167 = control-ref of="AScan"() -> (w561:refnum<vi>)
                  n168 = disable-structure shown="Enabled" {
                    disable-tunnel: w544 -> [w612 _]
                    disable-tunnel: w543 -> [w610 _]
                    frame Disabled {
                      n169 = case shown="True" "Boolean 2" {
                        tunnel: w612 -> [_ w615]
                        tunnel: w610 -> [_ w613]
                        frame False {
                        }
                        frame True {
                          n170 = Number To Decimal String(number=w613) -> (decimal integer string=w617:string)  [unwired: 1 in]
                          n171 = Concatenate Strings("C:\\OCTData\\Telesto_Disp_" ("string"), w617, ".srr" ("string")) -> (w618:string)
                          n172 = String To Path(string=w618) -> (path=w619:path)
                          n173 = call "export Raw Data.vi"("Export File"=w619, "Raw Data Export Format Selection"=Raw_Data_Export_Format_Selection."SRR (Spectral Radar Raw)", "Data in"=w615) -> ()  [unwired: 3 in, 2 out]
                        }
                      }
                    }
                    frame Enabled {
                    }
                  }
                  n174 = case shown="True" "Image field correction" {
                    tunnel: w568 -> [w630 w633]
                    tunnel: [w630 w632] -> w547
                    tunnel: w552 -> [_ w631]
                    frame False {
                    }
                    frame True {
                      n175 = disable-structure shown="Disabled" {
                        disable-tunnel: w633 -> [w637 w643]
                        disable-tunnel: [w636 w639] -> w632
                        disable-tunnel: w631 -> [w634 w640]
                        frame Disabled {
                          n176 = local read "Scan Pattern"() -> (w638:refnum<class "Scan Pattern.lvclass">)
                          n177 = local read "ImageField"() -> (w635:refnum<class "ImageField.lvclass">)
                          n178 = call "correct Image Field.vi"("error in (no error)"=w634, "ImageField in"=w635, "Data in"=w637, "Scan Pattern in"=w638) -> ("Data out"=w636:refnum<class "Data.lvclass">)  [unwired: 3 out]
                        }
                        frame Enabled {
                          n179 = local read "GalvoControl"() -> (w642:refnum<class "Probe.lvclass">)
                          n180 = local read "Scan Pattern"() -> (w641:refnum<class "Scan Pattern.lvclass">)
                          n181 = call "correct B-Scan from Probe.vi"("error in (no error)"=w640, "Probe in"=w642, "Data in"=w643, "Scan Pattern in"=w641) -> ("Data out"=w639:refnum<class "Data.lvclass">)  [unwired: 3 out]
                        }
                      }
                    }
                  }
                  n182 = case shown="False" "Filter" {
                    tunnel: w547 -> [w621 w623]
                    tunnel: [w621 w622] -> w546
                    frame False {
                    }
                    frame True {
                      n183 = call "Filter Bank.vi"("Data in"=w623) -> ("Data out"=w622:refnum<class "Data.lvclass">)  [unwired: 6 in]
                    }
                  }
                  n184 = call-poly "display Data.vi"("error in (no error)"=w552, "Index of Refraction"=w570, "Data in"=w546, "IntGraph Refnum"=w580) -> ("error out"=w566:errorcluster, "Data out"=w578:refnum<class "Data.lvclass">)  [unwired: 1 in, 1 out]
                  n185 = Merge Errors(w567, w566) -> (w564:errorcluster)
                  n186 = Merge Errors(w565, w564) -> (w571:errorcluster)
                  n187 = case shown="True" "ShowVideoImage" {
                    tunnel: w588 -> [_ w655]
                    tunnel: w571 -> [_ w647]
                    tunnel: [_ w649] -> w553
                    frame False {
                    }
                    frame True {
                      n188 = call "create Colored Data.vi"() -> ("error out"=w648:errorcluster, "Colored Data"=w654:refnum<class "Colored Data.lvclass">)  [unwired: 6 in]
                      n189 = Merge Errors(w648, w647) -> (w646:errorcluster)
                      n190 = call "get Camera Image.vi"("error in (no error)"=w646, "Colored Data in"=w654, "OCTDevice in"=w655) -> ("error out"=w650:errorcluster, "Colored Data out"=w644:refnum<class "Colored Data.lvclass">)  [unwired: 4 in, 1 out]
                      n191 = local read "Image"() -> (w652:T3)
                      n192 = call "update Colored Data IMAQ Image.vi"("error in (no error)"=w650, "Image in"=w652, "Colored Data"=w644) -> ("error out"=w651:errorcluster, "Image out"=→"Image":T3, "Colored Data"=w649:refnum<class "Colored Data.lvclass">)  [unwired: 2 in]
                      n193 = Unbundle By Name(w651) -> ("status"=w645:bool)
                      n194 = call <vilib>:"Simple Error Handler.vi"("error in (no error)"=w651) -> ()  [unwired: 4 in, 5 out]
                      n195 = case shown="True" w645 {
                        tunnel: w645 -> [_ w657]
                        frame False {
                        }
                        frame True {
                          n196 = Not(x=w657) -> (.not. x?=w656:bool)
                          n197 = local write "ShowVideoImage"(w656) -> ()
                        }
                      }
                    }
                  }
                  n198 = Unbundle By Name(w564) -> ("status"=w589:bool)
                  n199 = case shown="True" "Average A-scan" {
                    tunnel: w578 -> [w603 w609]
                    tunnel: w563 -> [w602 w608]
                    tunnel: [w601 w604] -> w562
                    tunnel: w560 -> [w600 _]
                    tunnel: Normal_Direction_Selection."Direction 2" ("Normal Direction") -> [w599 w607]
                    tunnel: [w598 w605] -> w554
                    frame False {
                      n200 = call "get Data Slice Index.vi"("Normal Direction"=w599, "Index"=w600, "Slice"=w602, "Data"=w603) -> ("Slice"=w601:refnum<class "Data.lvclass">, "Data"=w598:refnum<class "Data.lvclass">)  [unwired: 3 in, 1 out]
                    }
                    frame True {
                      n201 = call "get Data Slice Analyzed.vi"("Normal Direction"=w607, "Data Analyzation Selection"=Data_Analyzation_Selection."Mean", "Slice"=w608, "Data"=w609) -> ("Slice"=w604:refnum<class "Data.lvclass">, "Data"=w605:refnum<class "Data.lvclass">)  [unwired: 3 in, 1 out]
                    }
                  }
                  n202 = Compound Arithmetic op=OR(w589, w593, w585, w586) -> (w592:bool)
                  n203 = call-poly "display Data.vi"("Data"=w562, "XYGraph Refnum"=w561) -> ("Data"=w556:refnum<class "Data.lvclass">)  [unwired: 2 in, 3 out]
                  n204 = call "clear Data.vi"("Data"=w556) -> ()  [unwired: 6 in, 1 out]
                  n205 = case shown="False" "Auto Range Button" {
                    tunnel: w554 -> [w624 w629]
                    tunnel: [w624 w628] -> w540
                    frame False {
                    }
                    frame True {
                      n206 = call "determine Dynamic Range.vi"("Data in"=w629) -> ("High"=w627:sgl, "Low"=w626:sgl, "Data out"=w628:refnum<class "Data.lvclass">)  [unwired: 3 in, 1 out]
                      n207 = Bundle("High"=w627, "Low"=w626) -> (w625:cluster{"High":sgl, "Low":sgl})  [unwired: 1 in]
                      n208 = property on="Boundries" class="Slide (strict)"("Val(Sgnl)"=w625) -> ()  [unwired: 2 in, 2 out]
                    }
                  }
                  n209 = call "append to Buffer.vi"("Colored Data"=w553, "Data"=w540, "Buffer in"=w576) -> ("error out"=w573:errorcluster, "Buffer out"=w575:refnum<class "Buffer.lvclass">)  [unwired: 3 in]
                  n210 = call "get Buffer Size.vi"("error in (no error)"=w573, "Buffer in"=w575) -> ("Buffer Size"=w572:i32, "Buffer out"=w574:refnum<class "Buffer.lvclass">)  [unwired: 3 in, 1 out]
                  n211 = local write "Image#"(w572) -> ()
                }
                n212 = call <vilib>:"Set Busy.vi"("error in (no error)"=w506) -> ("error out"=w517:errorcluster)  [unwired: 9 in, 1 out]
                n213 = call "get Buffer Size.vi"("error in (no error)"=w506, "Buffer in"=w512) -> ("Buffer Size"=w510:i32, "Buffer out"=w511:refnum<class "Buffer.lvclass">)  [unwired: 3 in, 1 out]
                n214 = call "clear Raw Data.vi"("Raw Data"=w509) -> ()  [unwired: 6 in, 1 out]
                n215 = call "activate Standby.vi"("StandBy"=w519, "OCTDevice"=w505) -> ()  [unwired: 4 in, 2 out]
                n216 = local read "Scan Pattern"() -> (w507:refnum<class "Scan Pattern.lvclass">)
                n217 = Number To Decimal String(number=w510) -> (decimal integer string=w524:string)  [unwired: 1 in]
                n218 = property on="Image#" class="DigNum (strict)"("Maximum"=w510, "Minimum"=1.0 ("Data Entry Limits:Minimum")) -> ()  [unwired: 2 in, 2 out]
                n219 = call "clear Scan Pattern.vi"("error in (no error)"=w506, "Scan Pattern in"=w507) -> ()  [unwired: 5 in, 1 out]
                n220 = call "stop Measurement.vi"("OCTDevice"=w505) -> ("OCTDevice"=w521:refnum<class "OCT Device.lvclass">)  [unwired: 5 in, 1 out]
                n221 = Greater Than 0?(x=w510) -> (x > 0?=w528:bool)
                n222 = Greater?(x=w510, y=1) -> (0:w526:bool)
                n223 = Concatenate Strings("of " ("String"), w524) -> (w523:string)
                n224 = property on="Image#" class="DigNum (strict)"(error in=w506, "Caption.Visible"=TRUE ("Untertitel.Sichtbar")) -> ()  [unwired: 1 in, 2 out]
                n225 = flat-sequence {
                  tunnel: w528 -> [w535]
                  tunnel: w526 -> [w534]
                  tunnel: w517 -> [w532]
                  frame #0 {
                    w531 = u8 0 ("Deaktiviert")
                    n226 = case shown="True" w535 {
                      tunnel: w531 -> [_ w536]
                      frame False {
                      }
                      frame True {
                        n227 = property on="Save" class="Bool"("Disabled"=w536) -> ()  [unwired: 2 in, 2 out]
                        n228 = property on="Save all" class="Bool (strict)"("Disabled"=w536) -> ()  [unwired: 2 in, 2 out]
                      }
                    }
                    n229 = case shown="True" w534 {
                      tunnel: w531 -> [_ w537]
                      frame False {
                      }
                      frame True {
                        n230 = property on="Image#" class="DigNum (strict)"("Disabled"=w537) -> ()  [unwired: 2 in, 2 out]
                      }
                    }
                    n231 = property on="Range X [mm]" class="DigNum (strict)"(error in=w532, "Disabled"=w531) -> ()  [unwired: 1 in, 2 out]
                    n232 = property on="Averaging*Binning" class="Slide (strict)"("Disabled"=w531) -> ()  [unwired: 2 in, 2 out]
                    n233 = property on="Columns" class="DigNum (strict)"("Disabled"=w531) -> ()  [unwired: 2 in, 2 out]
                    n234 = property on="Recallibrate" class="Bool"("Disabled"=w531) -> ()  [unwired: 2 in, 2 out]
                    n235 = property on="Stability" class="Slide (strict)"("Disabled"=w531) -> ()  [unwired: 2 in, 2 out]
                    n236 = property on="BScan\nX offset [mm]" class="DigNum (strict)"("DisabledEnum"=w531) -> ()  [unwired: 2 in, 2 out]
                    n237 = property on="BScan\nY offset [mm]" class="DigNum (strict)"("DisabledEnum"=w531) -> ()  [unwired: 2 in, 2 out]
                    n238 = property on="BScan angle \n[deg]" class="Knob (strict)"("DisabledEnum"=w531) -> ()  [unwired: 2 in, 2 out]
                    n239 = property on="Streaming" class="Bool (strict)"("Disabled"=u8 0 ("Deaktiviert")) -> ()  [unwired: 2 in, 2 out]
                  }
                }
                n240 = property on="Image#" class="DigNum (strict)"(error in=w506, "Caption.Text"=w523) -> ()  [unwired: 1 in, 2 out]
                n241 = call <vilib>:"Unset Busy.vi"("error in (no error)"=w517) -> ()  [unwired: 10 in, 1 out]
                n242 = flat-sequence {
                  tunnel: w517 -> [_]
                  frame #0 {
                    n243 = local write "RunMeasurement"(FALSE ("StopIndicator")) -> ()
                    n244 = local write "StopIndicator"(FALSE ("StopIndicator")) -> ()
                  }
                }
              }
              frame Error {
                w659 = T16."Enabled" ("Disabled")
                w663 = FALSE ("RunMeasurement")
                n245 = local write "RunMeasurement"(w663) -> ()
                n246 = local write "StopIndicator"(w663) -> ()
                n247 = call "stop Measurement.vi"("OCTDevice"=w662) -> ("OCTDevice"=w661:refnum<class "OCT Device.lvclass">)  [unwired: 5 in, 1 out]
                n248 = property on="Stability" class="Slide (strict)"("DisabledEnum"=w659) -> ()  [unwired: 2 in, 2 out]
                n249 = property on="Averaging*Binning" class="Slide (strict)"("DisabledEnum"=w659) -> ()  [unwired: 2 in, 2 out]
              }
            }
          }
        }
        n250 = call <vilib>:"Simple Error Handler.vi"("error in (no error)"=w461) -> ()  [unwired: 4 in, 5 out]
      }
      n251 = while {
        tunnel: w175 -> [w179]
        tunnel: w172 -> [w178]
        tunnel: w169 -> [w177]
        stop <- w181 stop-if-true
        n252 = event shown="[2] \"Averaging*Binning\", \"Columns\", \"Range X [mm]\", \"Stability\": Value Change" {
          selector: _ -> [_ _ _ _ _ _ _ _ _ _ _ _ _ _ _ _ _ _ _ _]
          dyn-events: _ -> [_ _ _ _ _ _ _ _ _ _ _ _ _ _ _ _ _ _ _ _]
          timeout: 1000 -> [_ _ _ _ _ _ _ _ _ _ _ _ _ _ _ _ _ _ _ _]
          tunnel: w179 -> [w182 w185 _ _ w220 w227 w231 _ _ _ w289 _ _ _ _ _ w378 w396 _ _]
          tunnel: w178 -> [_ w184 w196 w216 w221 _ _ _ _ _ w288 w336 _ _ _ _ _ w395 _ _]
          tunnel: w177 -> [_ _ _ _ _ _ w230 w253 _ _ w287 _ _ _ _ w377 _ w394 _ _]
          event Timeout {
            n253 = event-data() -> ()  [unwired: 1 in, 1 out]
            n254 = call "check for Standby.vi"() -> ("TimeOut"=w183:bool)  [unwired: 1 in, 1 out]
            n255 = call "activate Standby.vi"("StandBy"=w183, "OCTDevice"=w182) -> ()  [unwired: 4 in, 2 out]
          }
          event "Recallibrate": Value Change {
            n256 = event-data() -> ()  [unwired: 1 in, 1 out]
            n257 = case shown="True" "Recallibrate" {
              tunnel: w185 -> [_ w191]
              tunnel: w184 -> [_ w192]
              frame False {
              }
              frame True {
                n258 = call "calibrate.vi"("Camera index"=0, "Processing in"=w192, "OCTDevice"=w191) -> ("error out"=w189:errorcluster, "OCTDevice"=w190:refnum<class "OCT Device.lvclass">)  [unwired: 2 in, 1 out]
                n259 = local read "GalvoControl"() -> (w194:refnum<class "Probe.lvclass">)
                n260 = call "close Probe.vi"("error in (no error)"=w189, "GalvoControl"=w194) -> ("error out"=w193:errorcluster)  [unwired: 5 in]
                n261 = call "init Probe.vi"("error in (no error)"=w193, "OCT Device [In]"=w190) -> ("GalvoControl"=w187:refnum<class "Probe.lvclass">)  [unwired: 3 in, 2 out]
                n262 = local write "GalvoControl"(w187) -> ()
              }
            }
          }
          event "Averaging*Binning", "Columns", "Range X [mm]", "Stability": Value Change {
            n263 = event-data() -> ()  [unwired: 1 in, 1 out]
            n264 = Decrement(x="Averaging*Binning") -> (x-1=w200:i32)
            n265 = Multiply(x=w200, y="Stability") -> (x*y=w203:dbl)
            n266 = local read "GalvoControl"() -> (w195:refnum<class "Probe.lvclass">)
            n267 = To Long Integer(number=w203) -> (32bit integer=w202:i32)
            n268 = Increment(x=w200) -> (x+1=w201:i32)
            n269 = Increment(x=w202) -> (x+1=w198:i32)
            n270 = Quotient & Remainder(x=w201, y=w198) -> (floor(x/y)=w199:i32)  [unwired: 1 out]
            n271 = disable-structure shown="Enabled" {
              disable-tunnel: w195 -> [w215 _]
              disable-tunnel: w199 -> [w213 _]
              disable-tunnel: w198 -> [w210 _]
              disable-tunnel: "Averaging*Binning" -> [w209 _]
              disable-tunnel: w196 -> [w207 _]
              frame Enabled {
                n272 = call "set Probe Parameter Int.vi"("Value"=w209, "Probe Parameter Int"=Probe_Parameter_Int_Selection."Oversampling", "GalvoControl"=w215) -> ("error out"=w208:errorcluster)  [unwired: 3 in, 1 out]
                n273 = call "set Processing Parameter Int.vi"("error in (no error)"=w208, "Value"=w213, "Processing Paramter Int Selection"=Processing_Parameter_Int_Selection."Spectrum Averaging", "Processing in"=w207) -> ("error out"=w211:errorcluster, "Processing out"=w206:refnum<class "Processing.lvclass">)  [unwired: 2 in]
                n274 = call "set Processing Parameter Int.vi"("error in (no error)"=w211, "Value"=w210, "Processing Paramter Int Selection"=Processing_Parameter_Int_Selection."A-Scan Averaging", "Processing in"=w206) -> ()  [unwired: 2 in, 2 out]
              }
              frame Disabled {
              }
            }
          }
          event "B-Scan \nAveraging": Value Change {
            n275 = event-data() -> ()  [unwired: 1 in, 1 out]
            n276 = call "set Processing Parameter Int.vi"("Value"="B-Scan \nAveraging", "Processing Paramter Int Selection"=Processing_Parameter_Int_Selection."B-Scan Averaging", "Processing in"=w216) -> ()  [unwired: 3 in, 2 out]
          }
          event "Options": Value Change {
            n277 = event-data() -> ()  [unwired: 1 in, 1 out]
            n278 = local read "GalvoControl"() -> (w219:refnum<class "Probe.lvclass">)
            n279 = case shown="True" "Options" {
              tunnel: w221 -> [_ w225]
              tunnel: w220 -> [_ w224]
              tunnel: w219 -> [_ w223]
              frame False {
              }
              frame True {
                n280 = call "Options Dialog.vi"("GalvoControl"=w223, "Processing"=w225, "OCT Device"=w224) -> ()  [unwired: 1 in]
              }
            }
          }
          event "Light": Value Change {
            n281 = event-data() -> ()  [unwired: 1 in, 1 out]
            n282 = call "set Output Device Value by Name.vi"("Value"="Light", "Identifier"="ring light", "OCTDevice"=w227) -> ("error out"=w226:errorcluster)  [unwired: 3 in, 1 out]
            n283 = call <vilib>:"Simple Error Handler.vi"("error in (no error)"=w226) -> ()  [unwired: 4 in, 5 out]
          }
          event "Index of Refraction": Value Change {
            n284 = event-data() -> ()  [unwired: 1 in, 1 out]
            n285 = flat-sequence {
              tunnel: w231 -> [w235]
              tunnel: w230 -> [_]
              frame #0 {
                n286 = call "get Device Property Float.vi"("Device Property Float Selection"=T5."z Range", "OCTDevice"=w235) -> ("Value"=w237:dbl)  [unwired: 3 in, 2 out]
                n287 = call "get Device Property Float.vi"("Device Property Float Selection"=T5."z Spacing", "OCTDevice"=w235) -> ("Value"=w233:dbl)  [unwired: 3 in, 2 out]
                n288 = Divide(x=w233, y="Index of Refraction") -> (x/y=w232:dbl)
                n289 = Divide(x=w237, y="Index of Refraction") -> (x/y=w240:dbl)
                n290 = Multiply(x=w240, y=0.2) -> (x*y=w244:dbl)
                n291 = property on="UpperBScanBorder" class="DigNum (strict)"("Wertebereich:Maximum"=w244) -> ()  [unwired: 2 in, 2 out]
                n292 = property on="AScan" class="XYGraph (strict)"("y-Achse.Offset und Faktor:Faktor"=w232) -> ()  [unwired: 2 in, 2 out]
                n293 = property on="B-Scan" class="IntGraph (strict)"("YScale.Multiplier"=w232) -> ()  [unwired: 2 in, 2 out]
                n294 = Multiply(x=w240, y=1.0) -> (x*y=w243:dbl)
                n295 = Multiply(x=w240, y=0.3) -> (x*y=w241:dbl)
                n296 = property on="LowerBScanBorder" class="DigNum (strict)"("Wertebereich:Maximum"=w243, "Minimum"=w241) -> ()  [unwired: 2 in, 2 out]
              }
              frame #1 {
                n297 = control-ref of="B-Scan"() -> (w250:refnum<vi>)
                n298 = control-ref of="AScan"() -> (w249:refnum<vi>)
                n299 = call "Cursors.vi"("Cursors"="Cursors", "IndexOfRefraction"=sgl 1.0, "ReferenceAScan"=w249, "ReferenceBScan"=w250) -> ("DistanceZ"=→"Distance Y [mm]":sgl, "DistanceX"=→"Distance X [mm]":sgl)
              }
            }
          }
          event "B-Scan": Cursor Move; "Cursors": Value Change {
            n300 = event-data() -> ()  [unwired: 1 in, 4 out]
            n301 = control-ref of="B-Scan"() -> (w273:refnum<vi>)
            n302 = control-ref of="AScan"() -> (w272:refnum<vi>)
            n303 = local read "Cursors"() -> (w269:bool)
            "Cursor on" <- w269
            n304 = call "Cursors.vi"("Cursors"=w269, "IndexOfRefraction"=sgl 1.0, "ReferenceAScan"=w272, "ReferenceBScan"=w273) -> ("DistanceZ"=w270:sgl, "DistanceX"=w271:sgl)
            n305 = local write "Distance X [mm]"(w271) -> ()
            n306 = local write "Distance Y [mm]"(w270) -> ()
            n307 = local read "Image#"() -> (w254:i32)
            n308 = Decrement(x=w254) -> (x-1=w255:i32)
            n309 = control-ref of="B-Scan"() -> (w267:refnum<vi>)
            n310 = call "get Buffer Data.vi"("Index"=w255, "Buffer in"=w253) -> ("Data out"=w268:refnum<class "Data.lvclass">)  [unwired: 3 in, 2 out]
            n311 = call "get Colored Buffer Data.vi"("Index"=w255, "Buffer in"=w253) -> ("Colored Data"=w266:refnum<class "Colored Data.lvclass">)  [unwired: 3 in, 2 out]
            n312 = call-poly "display Data.vi"("Data in"=w268, "IntGraph Refnum"=w267) -> ("Data out"=w262:refnum<class "Data.lvclass">)  [unwired: 3 in, 2 out]
            n313 = call "colored Data to IMAQ Image.vi"("Colored Data"=w266) -> ("Image Out"=w265:T3)  [unwired: 4 in, 2 out]
            n314 = local write "Image"(w265) -> ()
            n315 = call "create Data.vi"() -> ("Data"=w263:refnum<class "Data.lvclass">)  [unwired: 6 in, 1 out]
            n316 = property on="B-Scan" class="IntGraph (strict)"() -> ("Cursor.Cursor X"=w258:dbl, "XScale.Multiplier"=w257:dbl)  [unwired: 2 in, 2 out]
            n317 = Divide(x=w258, y=w257) -> (x/y=w256:dbl)
            n318 = call "get Data Slice Index.vi"("Normal Direction"=Normal_Direction_Selection."Direction 2", "Index"=w256, "Slice"=w263, "Data"=w262) -> ("Slice"=w261:refnum<class "Data.lvclass">)  [unwired: 3 in, 2 out]
            n319 = control-ref of="AScan"() -> (w260:refnum<vi>)
            n320 = call-poly "display Data.vi"("Orientation"=enum16{"Horizontal", "Vertical"}."Vertical", "Data"=w261, "XYGraph Refnum"=w260) -> ("Data"=w259:refnum<class "Data.lvclass">)  [unwired: 1 in, 3 out]
            n321 = call "clear Data.vi"("Data"=w259) -> ()  [unwired: 6 in, 1 out]
          }
          event "Boundries": Value Change {
            n322 = event-data() -> ()  [unwired: 1 in, 1 out]
            n323 = local read "Coloring"() -> (w279:refnum<class "Coloring.lvclass">)
            n324 = local read "Palette"() -> (w281:T1)
            n325 = call "clear Coloring.vi"("Coloring"=w279) -> ("error out"=w276:errorcluster)  [unwired: 6 in]
            n326 = control-ref of="B-Scan"() -> (w285:refnum<vi>)
            n327 = call "create Coloring.vi"("error in (no error)"=w276, "Color Byte Order"=Coloring_Byteorder."RGBA32", "Color Table Selection"=w281) -> ("error out"=w277:errorcluster, "Coloring"=w280:refnum<class "Coloring.lvclass">)  [unwired: 3 in]
            n328 = call "Palette Graph.vi"("Reference to the B-scan Graph"=w285, "Boundaries"="Boundries", "Color Scheme"=w281) -> ()
            n329 = Unbundle("Boundries") -> (w282:sgl, w283:sgl)
            n330 = property on="AScan" class="XYGraph (strict)"("XScale.Maximum"=w282, "XScale.Minimum"=w283) -> ()  [unwired: 2 in, 2 out]
            n331 = call "set Coloring Boundaries.vi"("error in (no error)"=w277, "Danymic Range High [dB]"=w282, "Dynamic Range Low [dB]"=w283, "Coloring in"=w280) -> ("Coloring out"=w278:refnum<class "Coloring.lvclass">)  [unwired: 2 in, 1 out]
            n332 = local write "Coloring"(w278) -> ()
          }
          event "Filter Options": Value Change {
            n333 = event-data() -> ()  [unwired: 1 in, 1 out]
            n334 = case shown="True" "Filter Options" {
              frame False {
              }
              frame True {
                n335 = call "Filter Bank.vi"() -> ()  [unwired: 7 in, 1 out]
              }
            }
          }
          event "Save all": Value Change {
            n336 = event-data() -> ()  [unwired: 1 in, 1 out]
            n337 = case shown="True" "Save all" {
              tunnel: w289 -> [_ _]
              tunnel: w288 -> [_ _]
              tunnel: w287 -> [_ w302]
              frame False {
              }
              frame True {
                n338 = call "get Buffer Size.vi"("Buffer in"=w302) -> ("error out"=w296:errorcluster, "Buffer Size"=w301:i32)  [unwired: 4 in, 1 out]
                n339 = Decrement(x=w301) -> (x-1=w295:i32)
                n340 = local write "Save All Progress"(0 ("Save All Progress")) -> ()
                n341 = property on="Save All Progress" class="Slide (strict)"(error in=w296, "Scale.Maximum"=w295, "Minimum"=0.0 ("Data Entry Limits:Minimum")) -> (error out=w297:errorcluster)  [unwired: 1 in, 1 out]
                n342 = property on="Save All Progress" class="Slide (strict)"(error in=w297, "Visible"=TRUE) -> (error out=w293:errorcluster)  [unwired: 1 in, 1 out]
                n343 = local read "Coloring"() -> (w291:refnum<class "Coloring.lvclass">)
                n344 = for {
                  N: w301 -> [_]
                  tunnel: w302 -> [w316]
                  tunnel: w291 -> [w315]
                  tunnel: [FALSE ("Visible")] -> w298
                  shift-right: [w309] -> w292
                  shift-left: w293 -> [w307]
                  i -> [w312]
                  n345 = control-ref of="Next File Name"() -> ()  [unwired: 1 out]
                  n346 = Increment(x=w312) -> (x+1=w314:i32)
                  n347 = call "get Colored Buffer Data.vi"("error in (no error)"=w307, "Index"=w312, "Buffer in"=w316) -> ("error out"=w313:errorcluster, "Colored Data"=w323:refnum<class "Colored Data.lvclass">)  [unwired: 2 in, 1 out]
                  n348 = property on="Image#" class="DigNum (strict)"("Val(Sgnl)"=w314) -> ()  [unwired: 2 in, 2 out]
                  n349 = local read "Next File Name"() -> (w321:path)
                  n350 = Path To String(path=w321) -> (string=w320:string)
                  n351 = Concatenate Strings(w320, "_Video" ("name or relative path")) -> (w318:string)
                  n352 = String To Path(string=w318) -> (path=w317:path)
                  n353 = call "create Colored Data.vi"() -> ("Colored Data"=w329:refnum<class "Colored Data.lvclass">)  [unwired: 6 in, 1 out]
                  n354 = call "export Colored Data.vi"("error in (no error)"=w313, "File Name"=w317, "Colored Data Export Format Selection"=Colored_Data_Export_Format_Selection."JPG", "Colored Data in"=w323) -> ("error out"=w308:errorcluster)  [unwired: 2 in, 1 out]
                  n355 = call <vilib>:"Clear Errors.vi"("error in (no error)"=w308) -> ("error out"=w306:errorcluster)  [unwired: 5 in, 1 out]
                  n356 = call "get Buffer Data.vi"("error in (no error)"=w306, "Index"=w312, "Buffer in"=w316) -> ("error out"=w333:errorcluster, "Data out"=w334:refnum<class "Data.lvclass">)  [unwired: 2 in, 1 out]
                  n357 = call "export Data.vi"("error in (no error)"=w333, "Export File"=w321, "Data Export Format Selection"=Data_Export_Format_Selection."SRM (Spectral Radar Metafile)", "Data in"=w334) -> ("error out"=w331:errorcluster, "Data out"=w332:refnum<class "Data.lvclass">)  [unwired: 2 in]
                  n358 = call "export Data.vi"("error in (no error)"=w331, "Export File"=w321, "Data Export Format Selection"=Data_Export_Format_Selection."TXT", "Data in"=w332) -> ("error out"=w328:errorcluster, "Data out"=w330:refnum<class "Data.lvclass">)  [unwired: 2 in]
                  n359 = call "colorize Data.vi"("error in (no error)"=w328, "Colored Data"=w329, "Data"=w330, "Coloring in"=w315) -> ("error out"=w325:errorcluster, "Colored Data"=w327:refnum<class "Colored Data.lvclass">)  [unwired: 2 out]
                  n360 = call "export Colored Data.vi"("error in (no error)"=w325, "File Name"=w321, "Colored Data Export Format Selection"=Colored_Data_Export_Format_Selection."BMP", "Colored Data in"=w327) -> ("error out"=w310:errorcluster, "Colored Data out"=w324:refnum<class "Colored Data.lvclass">)  [unwired: 2 in]
                  n361 = call "clear Colored Data.vi"("Colored Data"=w324) -> ()  [unwired: 6 in, 1 out]
                  n362 = call "get Next Filename.vi"("error in (no error)"=w310) -> ("Next File Name"=w335:path, "error out"=w309:errorcluster)
                  n363 = local write "Next File Name"(w335) -> ()
                  "Save All Progress" <- w312
                }
                n364 = case shown="Error" w292 {
                  frame No Error {
                  }
                  frame Error {
                    n365 = One Button Dialog(message="Could not export \nthe data. Please \ncheck if the path \nis valid.") -> ()  [unwired: 1 in, 1 out]
                  }
                }
                n366 = property on="Save All Progress" class="Slide (strict)"("Visible"=w298) -> ()  [unwired: 2 in, 2 out]
              }
            }
          }
          event "Window": Value Change {
            n367 = event-data() -> ()  [unwired: 1 in, 6 out]
            n368 = call "set Apodization Window.vi"("Window"="Window", "Processing"=w336) -> ()  [unwired: 4 in, 2 out]
          }
          event "UpperBScanBorder", "LowerBScanBorder": Value Change {
            n369 = event-data() -> ()  [unwired: 1 in, 1 out]
            n370 = property on="B-Scan" class="IntGraph (strict)"("YScale.Minimum"="UpperBScanBorder", "YScale.Maximum"="LowerBScanBorder") -> ()  [unwired: 2 in, 2 out]
            n371 = property on="AScan" class="XYGraph (strict)"("YScale.Minimum"="UpperBScanBorder", "YScale.Maximum"="LowerBScanBorder") -> ()  [unwired: 2 in, 2 out]
          }
          event "QuitApp": Mouse Enter {
            n372 = event-data() -> ("Time"=w343:u32)  [unwired: 1 in]
            n373 = Tick Count (ms)() -> (millisecond timer value=w344:u32)
            n374 = Subtract(x=w344, y=w343) -> (x-y=w342:u32)
            n375 = Less?(x=w342, y=u32 200) -> (x < y?=w340:bool)
            n376 = case shown="True" w340 {
              frame False {
              }
              frame True {
                w345 = u32 16448250
                n377 = Bundle(u32 16711680, u32 16448250) -> (w347:cluster{u32, u32})  [unwired: 1 in]
                n378 = Bundle(u32 8978432, w345) -> (w346:cluster{u32, u32})  [unwired: 1 in]
                n379 = Build Array(w347, w346) -> (w349:cluster{u32, u32}[])
                n380 = property on="QuitApp" class="Bool (strict)"("Colors [4]"=w349, "BoolText.TextColor"=w345) -> ()  [unwired: 2 in, 2 out]
              }
            }
          }
          event "QuitApp": Mouse Leave {
            w352 = u32 0
            n381 = event-data() -> ()  [unwired: 1 in, 1 out]
            n382 = Bundle(u32 9868950, w352) -> (w353:cluster{u32, u32})  [unwired: 1 in]
            n383 = Bundle(u32 12369084, u32 0) -> (w354:cluster{u32, u32})  [unwired: 1 in]
            n384 = Build Array(w354, w353) -> (w358:cluster{u32, u32}[])
            n385 = property on="QuitApp" class="Bool (strict)"("Colors [4]"=w358, "BoolText.TextColor"=w352) -> ()  [unwired: 2 in, 2 out]
          }
          event "Image#": Value Change {
            n386 = event-data() -> ()  [unwired: 1 in, 1 out]
            n387 = Decrement(x="Image#") -> (x-1=w364:i32)
            n388 = call "get Buffer Data.vi"("Index"=w364, "Buffer in"=w377) -> ("Data out"=w375:refnum<class "Data.lvclass">)  [unwired: 3 in, 2 out]
            n389 = call "get Colored Buffer Data.vi"("Index"=w364, "Buffer in"=w377) -> ("Colored Data"=w363:refnum<class "Colored Data.lvclass">)  [unwired: 3 in, 2 out]
            n390 = local read "Index of Refraction"() -> (w360:dbl)
            n391 = control-ref of="B-Scan"() -> (w374:refnum<vi>)
            n392 = local read "Image"() -> (w361:T3)
            n393 = call "update Colored Data IMAQ Image.vi"("Image in"=w361, "Colored Data"=w363) -> ("Image out"=w362:T3)  [unwired: 3 in, 2 out]
            n394 = call-poly "display Data.vi"("Index of Refraction"=w360, "Data in"=w375, "IntGraph Refnum"=w374) -> ("Data out"=w371:refnum<class "Data.lvclass">)  [unwired: 2 in, 2 out]
            n395 = local write "Image"(w362) -> ()
            n396 = call "create Data.vi"() -> ("Data"=w372:refnum<class "Data.lvclass">)  [unwired: 6 in, 1 out]
            n397 = property on="B-Scan" class="IntGraph (strict)"() -> ("Cursor.Cursor X"=w367:dbl, "XScale.Multiplier"=w366:dbl)  [unwired: 2 in, 2 out]
            n398 = Divide(x=w367, y=w366) -> (x/y=w365:dbl)
            n399 = call "get Data Slice Index.vi"("Normal Direction"=Normal_Direction_Selection."Direction 2", "Index"=w365, "Slice"=w372, "Data"=w371) -> ("Slice"=w370:refnum<class "Data.lvclass">)  [unwired: 3 in, 2 out]
            n400 = control-ref of="AScan"() -> (w369:refnum<vi>)
            n401 = call-poly "display Data.vi"("Orientation"=enum16{"Horizontal", "Vertical"}."Horizontal", "Data"=w370, "XYGraph Refnum"=w369) -> ("Data"=w368:refnum<class "Data.lvclass">)  [unwired: 1 in, 3 out]
            n402 = call "clear Data.vi"("Data"=w368) -> ()  [unwired: 6 in, 1 out]
          }
          event "Set Path": Value Change {
            n403 = event-data() -> ()  [unwired: 1 in, 1 out]
            n404 = case shown="True" "Set Path" {
              tunnel: w378 -> [_ _]
              frame False {
              }
              frame True {
                n405 = local read "Next File Name"() -> (w382:path)
                n406 = File Dialog(4:"SpectralRadar Measurement File" ("pattern label"), 5:"Select" ("button label"), 6:"*.srm" ("pattern"), 7:"Select SpectralRadar Measurement" ("Abfrage"), 9:"Measurement" ("Standardname"), 11:w382) -> (1:w380:bool, 3:w381:path)  [unwired: 1 in, 2 out]
                n407 = case shown="False" w380 {
                  tunnel: w381 -> [w390 _]
                  frame False {
                    n408 = Path To String(path=w390) -> (string=w389:string)
                    n409 = call "set Base Filename.vi"("Base"=w389) -> ("error out"=w391:errorcluster)  [unwired: 1 in]
                    n410 = call "get Next Filename.vi"("error in (no error)"=w391) -> ("Next File Name"=→"Next File Name":path)  [unwired: 1 out]
                  }
                  frame True {
                  }
                }
              }
            }
          }
          event "Save": Value Change {
            n411 = event-data() -> ()  [unwired: 1 in, 1 out]
            n412 = local read "Coloring"() -> (w392:refnum<class "Coloring.lvclass">)
            n413 = case shown="True" "Save" {
              tunnel: w396 -> [_ _]
              tunnel: w395 -> [_ _]
              tunnel: w394 -> [_ w424]
              tunnel: w392 -> [_ w420]
              tunnel: [_ w401] -> w393
              frame False {
              }
              frame True {
                # "No camera image available is not severe. Suppress."
                n414 = local read "Image#"() -> (w425:i32)
                n415 = Decrement(x=w425) -> (x-1=w430:i32)
                n416 = Increment(x=w425) -> (x+1=w422:i32)
                n417 = call "get Buffer Size.vi"("Buffer in"=w424) -> ("Buffer Size"=w423:i32)  [unwired: 4 in, 2 out]
                n418 = call "get Colored Buffer Data.vi"("Index"=w430, "Buffer in"=w424) -> ("error out"=w405:errorcluster, "Colored Data"=w412:refnum<class "Colored Data.lvclass">)  [unwired: 3 in, 1 out]
                n419 = Max & Min(x=w422, y=w423) -> (min(x,y)=w421:i32)  [unwired: 1 out]
                n420 = local read "Next File Name"() -> (w410:path)
                n421 = property on="Image#" class="DigNum (strict)"("Val(Sgnl)"=w421) -> ()  [unwired: 2 in, 2 out]
                n422 = Path To String(path=w410) -> (string=w409:string)
                n423 = Concatenate Strings(w409, "_Video" ("name or relative path")) -> (w407:string)
                n424 = String To Path(string=w407) -> (path=w406:path)
                n425 = call "create Colored Data.vi"() -> ("Colored Data"=w418:refnum<class "Colored Data.lvclass">)  [unwired: 6 in, 1 out]
                n426 = call "export Colored Data.vi"("error in (no error)"=w405, "File Name"=w406, "Colored Data Export Format Selection"=Colored_Data_Export_Format_Selection."JPG", "Colored Data in"=w412) -> ("error out"=w403:errorcluster)  [unwired: 2 in, 1 out]
                n427 = call <vilib>:"Clear Errors.vi"("error in (no error)"=w403) -> ("error out"=w402:errorcluster)  [unwired: 5 in, 1 out]
                n428 = call "get Buffer Data.vi"("error in (no error)"=w402, "Index"=w430, "Buffer in"=w424) -> ("error out"=w428:errorcluster, "Data out"=w429:refnum<class "Data.lvclass">)  [unwired: 2 in, 1 out]
                n429 = call "export Data.vi"("error in (no error)"=w428, "Export File"=w410, "Data Export Format Selection"=Data_Export_Format_Selection."SRM (Spectral Radar Metafile)", "Data in"=w429) -> ("error out"=w426:errorcluster, "Data out"=w427:refnum<class "Data.lvclass">)  [unwired: 2 in]
                n430 = call "export Data.vi"("error in (no error)"=w426, "Export File"=w410, "Data Export Format Selection"=Data_Export_Format_Selection."TXT", "Data in"=w427) -> ("error out"=w417:errorcluster, "Data out"=w419:refnum<class "Data.lvclass">)  [unwired: 2 in]
                n431 = call "colorize Data.vi"("error in (no error)"=w417, "Colored Data"=w418, "Data"=w419, "Coloring in"=w420) -> ("error out"=w414:errorcluster, "Colored Data"=w416:refnum<class "Colored Data.lvclass">)  [unwired: 2 out]
                n432 = call "export Colored Data.vi"("error in (no error)"=w414, "File Name"=w410, "Colored Data Export Format Selection"=Colored_Data_Export_Format_Selection."BMP", "Colored Data in"=w416) -> ("error out"=w404:errorcluster, "Colored Data out"=w413:refnum<class "Colored Data.lvclass">)  [unwired: 2 in]
                n433 = call "clear Colored Data.vi"("Colored Data"=w413) -> ()  [unwired: 6 in, 1 out]
                n434 = call "get Next Filename.vi"("error in (no error)"=w404) -> ("Next File Name"=w431:path, "error out"=w401:errorcluster)
                n435 = local write "Next File Name"(w431) -> ()
              }
            }
            n436 = case shown="Error" w393 {
              frame No Error {
              }
              frame Error {
                n437 = One Button Dialog(message="Could not export \nthe data. Please \ncheck if the path \nis valid.") -> ()  [unwired: 1 in, 1 out]
              }
            }
          }
          event Mouse Down; Mouse Up {
            n438 = event-data() -> ()  [unwired: 1 in, 1 out]
            n439 = call "check for Standby.vi"("ResetTimer"=TRUE) -> ()  [unwired: 2 out]
          }
          event "AScan": Cursor Move {
            n440 = event-data() -> ()  [unwired: 1 in, 1 out]
            n441 = property on="AScan" class="XYGraph (strict)"("Active Cursor"=u32 0 ("Aktiver Cursor"), "Active Cursor"=u32 1 ("Aktiver Cursor")) -> ("Cursor.Cursor Y"=w442:dbl, "Cursor.Cursor Y"=w441:dbl)  [unwired: 2 in, 2 out]
            n442 = property on="B-Scan" class="IntGraph (strict)"("Active Cursor"=u32 0 ("Aktiver Cursor"), "Cursor.Cursor Y"=w442, "Active Cursor"=u32 1 ("Aktiver Cursor"), "Cursor.Cursor Y"=w441) -> ()  [unwired: 2 in, 2 out]
            n443 = local read "Index of Refraction"() -> (w438:dbl)
            n444 = control-ref of="B-Scan"() -> (w433:refnum<vi>)
            n445 = control-ref of="AScan"() -> (w437:refnum<vi>)
            n446 = local read "Cursors"() -> (w436:bool)
            n447 = call "Cursors.vi"("Cursors"=w436, "IndexOfRefraction"=w438, "ReferenceAScan"=w437, "ReferenceBScan"=w433) -> ("DistanceZ"=w434:sgl, "DistanceX"=w435:sgl)
            n448 = local write "Distance X [mm]"(w435) -> ()
            n449 = local write "Distance Y [mm]"(w434) -> ()
            n450 = local write "Cursor on"(w436) -> ()
          }
        }
        n451 = local read "QuitApp"() -> (w181:bool)
      }
    }
    frame #4 {
      n452 = local read "ImageField"() -> (w664:refnum<class "ImageField.lvclass">)
      n453 = local read "Coloring"() -> (w665:refnum<class "Coloring.lvclass">)
      n454 = call "clear Processing.vi"("Processing"=w667) -> ()  [unwired: 6 in, 1 out]
      n455 = call "clear Buffer.vi"("Buffer"=w666) -> ()  [unwired: 6 in, 1 out]
      n456 = call "clear Coloring.vi"("Coloring"=w665) -> ()  [unwired: 6 in, 1 out]
      n457 = call "clear Image Field.vi"("ImageField in"=w664) -> ()  [unwired: 6 in, 1 out]
    }
    frame #5 {
      n458 = call "close Device.vi"("OCTDevice"=w669) -> ()  [unwired: 6 in, 1 out]
    }
    frame #6 {
      n459 = local read "AutoSafe"() -> (w670:bool)
      n460 = case shown="True" w670 {
        frame False {
        }
        frame True {
          n461 = local read "Index of Refraction"() -> (w694:dbl)
          n462 = call "get Config Path.vi"() -> ("Path"=w672:path)  [unwired: 1 in, 1 out]
          n463 = local read "Range X [mm]"() -> (w692:dbl)
          n464 = local read "Saturation"() -> (w683:sgl)
          n465 = local read "Brightness"() -> (w680:sgl)
          n466 = local read "Columns"() -> (w696:i32)
          n467 = local read "Contrast"() -> (w679:sgl)
          n468 = local read "Window"() -> (w687:T2)
          n469 = local read "Palette"() -> (w671:T1)
          n470 = Build Path(base path=w672, name or relative path=path "Settings.ini" ("Relative \"SpectralRadar.ini\" Path")) -> (appended path=w698:path)
          n471 = call "init Settings.vi"("Path to settings file"=w698) -> ("Settings"=w691:refnum<class "Settings.lvclass">)  [unwired: 5 in, 1 out]
          n472 = call "set Settings Entry Int.vi"("Value"=w696, "Node"="Columns" ("Node Name"), "Settings"=w691) -> ("Settings"=w690:refnum<class "Settings.lvclass">)  [unwired: 3 in, 1 out]
          n473 = call "set Settings Entry Float.vi"("Value"=w694, "Node"="IndexOfRefraction" ("Node Name"), "Settings"=w690) -> ("Settings"=w689:refnum<class "Settings.lvclass">)  [unwired: 3 in, 1 out]
          n474 = call "set Settings Entry Float.vi"("Value"=w692, "Node"="Range" ("Node Name"), "Settings"=w689) -> ("Settings"=w675:refnum<class "Settings.lvclass">)  [unwired: 3 in, 1 out]
          n475 = call "set Settings Entry Float.vi"("Value"=w683, "Node"="Saturation" ("Node Name"), "Settings"=w675) -> ("Settings"=w682:refnum<class "Settings.lvclass">)  [unwired: 3 in, 1 out]
          n476 = call "set Settings Entry Float.vi"("Value"=w680, "Node"="Brightness" ("Node Name"), "Settings"=w682) -> ("Settings"=w678:refnum<class "Settings.lvclass">)  [unwired: 3 in, 1 out]
          n477 = call "set Settings Entry Float.vi"("Value"=w679, "Node"="Contrast" ("Node Name"), "Settings"=w678) -> ("Settings"=w677:refnum<class "Settings.lvclass">)  [unwired: 3 in, 1 out]
          n478 = call "set Settings Entry Int.vi"("Value"=w687, "Node"="ApodizationWindow" ("Node Name"), "Settings"=w677) -> ("Settings"=w685:refnum<class "Settings.lvclass">)  [unwired: 3 in, 1 out]
          n479 = call "set Settings Entry Int.vi"("Value"=w671, "Node"="Palette" ("Node Name"), "Settings"=w685) -> ("Settings"=w674:refnum<class "Settings.lvclass">)  [unwired: 3 in, 1 out]
          n480 = call "save Settings.vi"("Settings"=w674) -> ("Settings"=w673:refnum<class "Settings.lvclass">)  [unwired: 5 in, 1 out]
          n481 = call "close Settings.vi"("Settings"=w673) -> ()  [unwired: 6 in, 1 out]
        }
      }
    }
  }
